vi "Find Subscript Text.vi"(10 "String":string) -> (1 "Subscript Text":string[](array[string]), 2 "Regular Text":string[](array[string]), 4 "interleaved array":string[](array[string]), 5 "concatenated string":string)   [LabVIEW 2012, in "String XControl.xctl"]
uses:
  String XControl.xctl
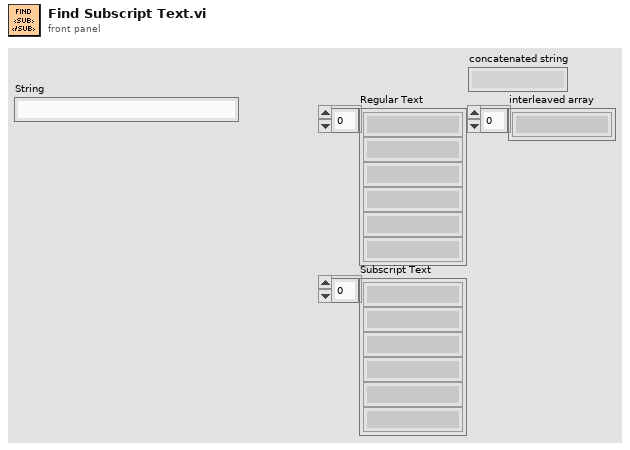
[diagram p1: front panel]
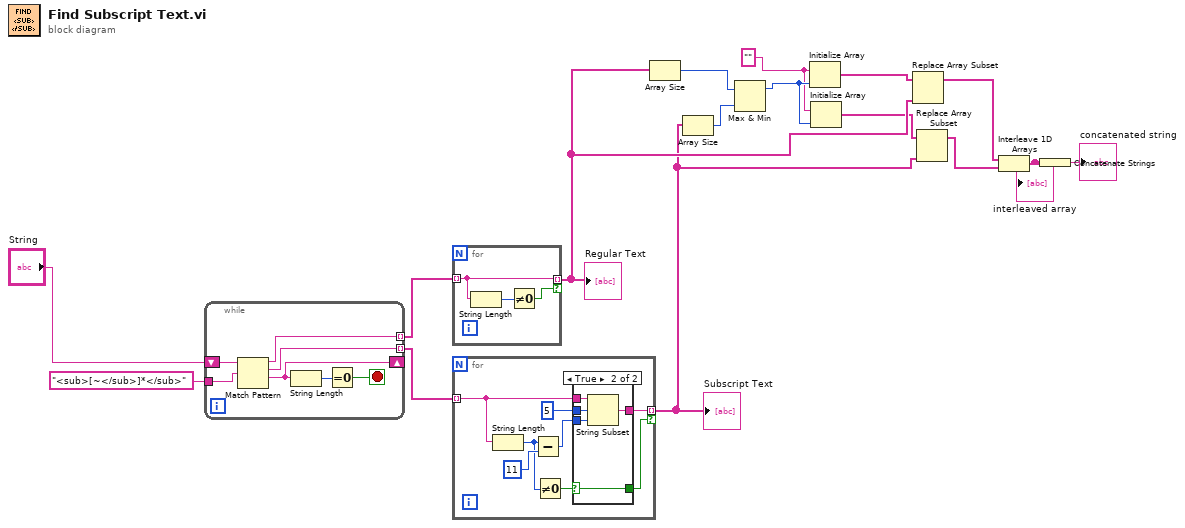
[diagram p0: block diagram]
diagram:
  w7 = "" ("concatenated string")
  n1 = while {
    shift-right: [w19] -> _
    shift-left: "String" -> [w23]
    tunnel: "<sub>[~</sub>]*</sub>" ("format string") -> [w22]
    tunnel: [w21] -> w14 mode=indexing
    tunnel: [w20] -> w13 mode=indexing
    stop <- w17 stop-if-true
    n2 = Match Pattern(string=w23, regular expression=w22) -> (before substring=w21:string, match substring=w20:string, after substring=w19:string)  [unwired: 1 in, 1 out]
    n3 = String Length(string=w19) -> (length=w18:i32)
    n4 = Equal To 0?(x=w18) -> (x = 0?=w17:bool)
  }
  n5 = for {
    tunnel: w14 -> [w25] mode=indexing
    tunnel: [w25] -> w5 mode=indexing if=w24
    n6 = String Length(string=w25) -> (length=w26:i32)
    n7 = Not Equal To 0?(x=w26) -> (x != 0?=w24:bool)
  }
  "Regular Text" <- w5
  n8 = for {
    tunnel: w13 -> [w33] mode=indexing
    tunnel: [w28] -> w2 mode=indexing if=w27
    n9 = String Length(string=w33) -> (length=w30:i32)
    n10 = Subtract(x=w30, y=11 ("offset (0)")) -> (x-y=w31:i32)
    n11 = Not Equal To 0?(x=w30) -> (x != 0?=w29:bool)
    n12 = case shown="True" w29 {
      selector: w29 -> [w35 w36]
      tunnel: 5 ("offset (0)") -> [_ w40]
      tunnel: w33 -> [_ w39]
      tunnel: w31 -> [_ w38]
      tunnel: [_ w37] -> w28
      tunnel: [w35 w36] -> w27
      frame False {
      }
      frame True {
        n13 = String Subset(string=w39, offset (0)=w40, length (rest)=w38) -> (substring=w37:string)
      }
    }
  }
  "Subscript Text" <- w2
  n14 = Array Size(array=w5) -> (size(s)=w9:i32)
  n15 = Array Size(array=w2) -> (size(s)=w10:i32)
  n16 = Max & Min(x=w9, y=w10) -> (max(x,y)=w8:i32)  [unwired: 1 out]
  n17 = Initialize Array(w7, w8) -> (w6:string[])
  n18 = Initialize Array(w7, w8) -> (w3:string[])
  n19 = Replace Array Subset(array=w6, new element=w5) -> (w4:string[])  [unwired: 1 in]
  n20 = Replace Array Subset(array=w3, new element=w2) -> (w1:string[])  [unwired: 1 in]
  n21 = Interleave 1D Arrays(w4, w1) -> (w12:string[])
  "interleaved array" <- w12
  n22 = Concatenate Strings(w12) -> (→"concatenated string":string)
